vi "Luminance_Pass_Filter.vi"(6 "Median Filter Size":dbl=3.0, 8 "Threshold Range":cluster{"Lower value":sgl, "Upper value":sgl}={"Lower value"=240.0, "Upper value"=255.0} {"Upper value" format="%.2f"; "Lower value" format="%.2f"}, 9 "Remove Dots Image Dst":T1, 10 "Filtered Image Dst":T1, 11 "Image Src":T1) -> (3 "Image Dst Out":T1)   [LabVIEW 2011]
uses:
  <vilib>/vision/Image Controls.llb/IMAQ Image.ctl
  <vilib>/vision/NI_Vision_Development_Module.lvlib
panel:
  in  "Replace Value":sgl=255.0 format="%.2f"
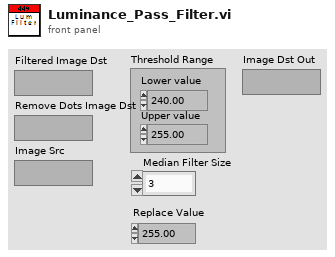
[diagram p1: front panel]
types:
  T1 = typedef "IMAQ Image.ctl" = refnum<image>
  T2 = cluster{"Median Filter Size":dbl, "Median Filter Size":dbl, dbl}
  T3 = cluster{"Median Filter Size":i32, "Median Filter Size":i32, i32}
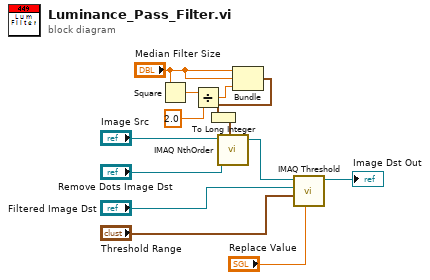
[diagram p0: block diagram]
diagram:
  n1 = Square(x="Median Filter Size") -> (x^2=w8:dbl)
  n2 = Divide(x=w8, y=2.0) -> (x/y=w6:dbl)
  n3 = Bundle("Median Filter Size"="Median Filter Size", "Median Filter Size"="Median Filter Size", w6) -> (w5:T2)  [unwired: 1 in]
  n4 = To Long Integer(number=w5) -> (32bit integer=w4:T3)
  n5 = call "IMAQ NthOrder"("Image Src"="Image Src", "Size & Order #"=w4, "Image Dst"="Remove Dots Image Dst") -> ("Image Dst Out"=w12:T1)  [unwired: 4 in, 1 out]
  n6 = call "IMAQ Threshold"("Replace Value"="Replace Value", "Range"="Threshold Range", "Image Dst"="Filtered Image Dst", "Image Src"=w12) -> ("Image Dst Out"=→"Image Dst Out":T1)  [unwired: 6 in, 1 out]
